vi "CloseDatabase.vi"(8 "error in (no error)":errorcluster, 11 "MongoDB-Database in":refnum<class "MongoDB-Database.lvclass">) -> (0 "error out":errorcluster)   [LabVIEW 2016, in "MongoDB-Database.lvlib" / "MongoDB-Database.lvclass"]
uses:
  MongoDB-Database.lvclass
  D:/Users/blume/Desktop/LV/MongoDB-Driver/MLV DLLs/MongoLabVIEW.dll
  LV/MongoDB-Driver/MLV DLLs/MongoLabVIEW.dll
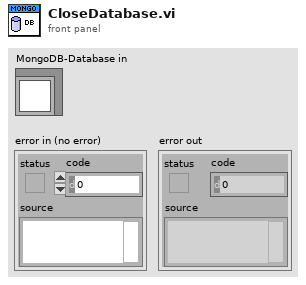
[diagram p1: front panel]
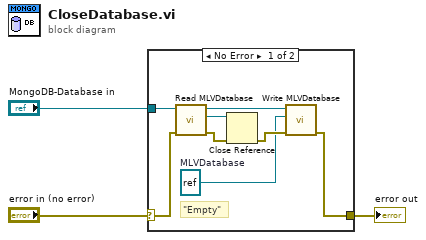
[diagram p0: block diagram]
diagram:
  n1 = case shown="No Error" "error in (no error)" {
    selector: "error in (no error)" -> [w4 w12]
    tunnel: [w5 w12] -> w2
    tunnel: "MongoDB-Database in" -> [w11 _]
    frame No Error {
      w6 = refnum<k24> refnum  # MLVDatabase
      # "\"Empty\""
      n2 = call "Read MLVDatabase.vi"("error in (no error)"=w4, "MongoDB-Database in"=w11) -> ("error out"=w9:errorcluster, "MLVDatabase"=w10:refnum<k24>, "MongoDB-Database out"=w8:refnum<class "MongoDB-Database.lvclass">)  [unwired: 7 in]
      n3 = Close Reference(reference=w10, error in (no error)=w9) -> (error out=w7:errorcluster)
      n4 = call "Write MLVDatabase.vi"("error in (no error)"=w7, "MLVDatabase"=w6, "MongoDB-Database in"=w8) -> ("error out"=w5:errorcluster)  [unwired: 7 in, 1 out]
    }
    frame Error {
    }
  }
  "error out" <- w2
